vi "Check For Type Mismatch Error.vi"(7 "Abs_Type":refnum<class "Abs_Type.lvclass">, 8 "error in (no error)":errorcluster, 11 "Abs_Value in":refnum<class "Abs_Value.lvclass">) -> (0 "error out":errorcluster, 3 "Abs_Value out":refnum<class "Abs_Value.lvclass">)   [LabVIEW 2021, in "Omni_Bus.lvclass"]
uses:
  Omni_Bus.lvclass
  <vilib>/TSA/Abstract Data Classes/Abs_Types/Value/Abs_Value.lvclass
  <vilib>/TSA/Abstract Data Classes/Abs_Types/Type/Abs_Type.lvclass
  <vilib>/Utility/error.llb/Error Cluster From Error Code.vi
  <vilib>/ErrorRing/Error Ring.xnode
  Omni_Bus.lvclass/Omni_Bus.ctl
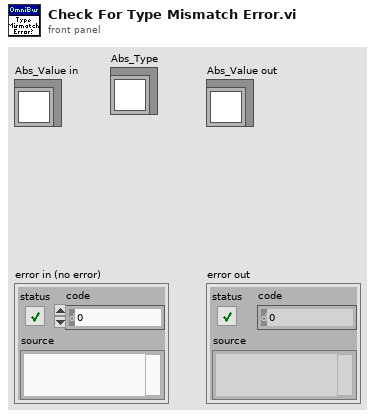
[diagram p1: front panel]
types:
  T1 = typedef "NI_Data Type.lvlib/Data Type.ctl" = enum8{"Invalid Type", "Void", "I8", "I16", "I32", "I64", "U8", "U16", "U32", "U64", "Single Float", "Double Float", "Extended Float", "Single Complex", "Double Complex", "Extended Complex", "Enum U8", "Enum U16", "Enum U32", "Enum U64", "Single Float With Unit", "Double Float With Unit", "Extended Float With Unit", "Single Complex with Unit", "Double Complex with Unit", "Extended Complex with Unit", "Boolean", "String", "Path", "Picture", "Tag", "Array", "Cluster", "Variant", "LV Variant", "Waveform", "Timestamp", "Digital Waveform", "Digital Data", "ExpressData", "Refnum", "External Data", "VI", "Poly VI", "LabVIEW Class Instance", "Fixed Point", "Set Collection", "Map Collection"}
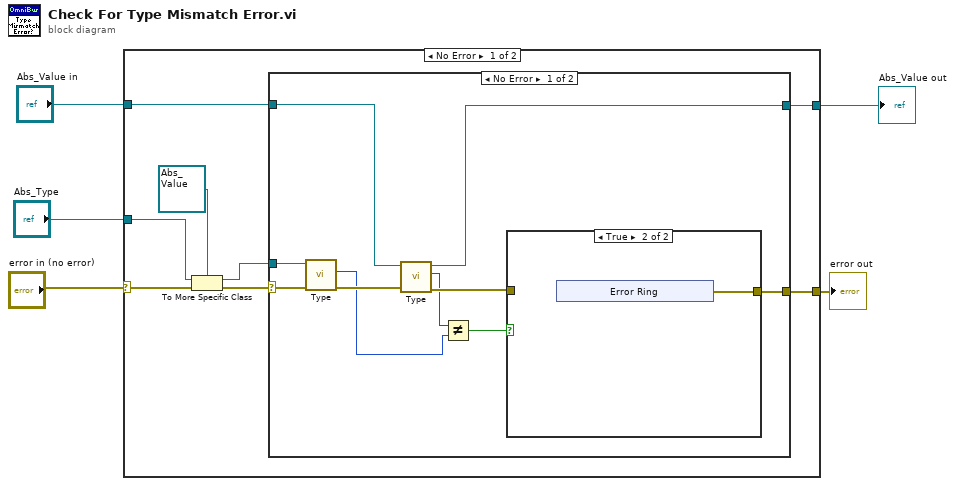
[diagram p0: block diagram]
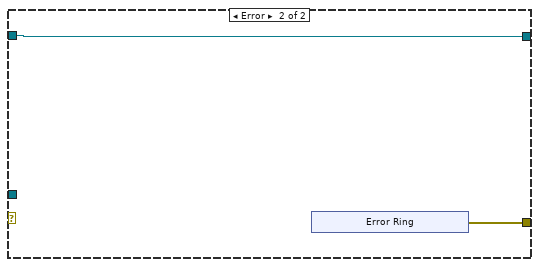
[diagram p3: hidden frame]
diagram:
  n1 = case shown="No Error" "error in (no error)" {
    selector: "error in (no error)" -> [w9 w38]
    tunnel: [w13 w38] -> w5
    tunnel: "Abs_Value in" -> [w12 w39]
    tunnel: [w11 w39] -> w3
    tunnel: "Abs_Type" -> [w7 _]
    frame No Error {
      n2 = To More Specific Class(target class=refnum<class "Abs_Value.lvclass"> refnum ("Abs_Value.lvclass"), reference=w7, error in=w9) -> (specific class reference=w6:refnum<class "Abs_Value.lvclass">, error out=w8:errorcluster)
      n3 = case shown="No Error" w8 {
        selector: w8 -> [w15 _]
        tunnel: [w23 w31] -> w13
        tunnel: w12 -> [w21 w32]
        tunnel: [w18 w32] -> w11
        tunnel: w6 -> [w14 _]
        frame No Error {
          n4 = call-dynamic "Type.vi"("error in (no error)"=w15, "Element in"=w14) -> ("error out"=w17:errorcluster, "Type"=w16:T1)  [unwired: 7 in, 1 out]
          n5 = call-dynamic "Type.vi"("error in (no error)"=w17, "Element in"=w21) -> ("error out"=w22:errorcluster, "Type"=w20:T1, "Element out"=w18:refnum<class "Abs_Value.lvclass">)  [unwired: 7 in]
          n6 = Not Equal?(x=w20, y=w16) -> (x != y?=w19:bool)
          n7 = case shown="True" w19 {
            tunnel: w22 -> [w24 _]
            tunnel: [w24 w25] -> w23
            frame False {
            }
            frame True {
              n8 = xnode "Error Ring"() -> ("error out"=w25:errorcluster)
            }
          }
        }
        frame Error {
          n9 = xnode "Error Ring"() -> ("error out"=w31:errorcluster)
        }
      }
    }
    frame Error {
    }
  }
  "error out" <- w5
  "Abs_Value out" <- w3
